vi "Update Value.vi"(6 "Time":dbl, 8 "error in (no error)":errorcluster, 11 "BooleanIndicator in":refnum<class "BooleanIndicator.lvclass">) -> (0 "error out":errorcluster, 1 "Update":bool, 2 "Value":variant, 3 "BooleanIndicator out":refnum<class "BooleanIndicator.lvclass">)   [LabVIEW 2020, in "VolatusGUIElements.lvlib" / "BooleanIndicator.lvclass"]
uses:
  BooleanIndicator.lvclass
  BooleanIndicator.lvclass/BooleanIndicator.ctl
  lv-vecto/Vecto/Channel DBL/Channel DBL.lvclass/Channel DBL.ctl
  lv-vecto/Vecto/Group DBL/Value by Index.vi
  lv-vecto/Vecto/Channel DBL/Channel DBL.lvclass
  lv-vecto/Vecto/Vecto.lvlib
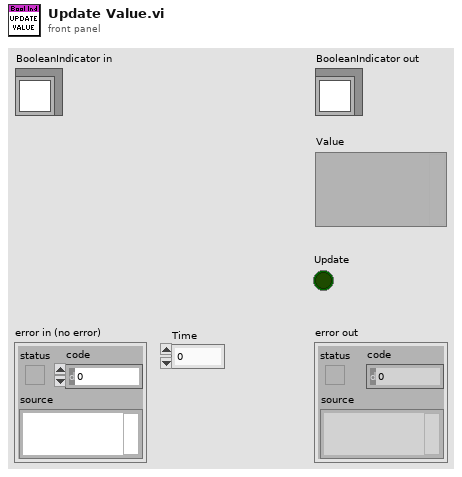
[diagram p1: front panel]
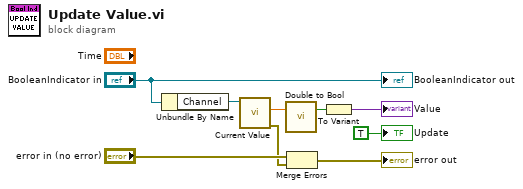
[diagram p0: block diagram]
diagram:
  n1 = Unbundle By Name("BooleanIndicator in") -> ("Channel"=w8:refnum<class "Channel DBL.lvclass">)
  n2 = call "Current Value.vi"("Channel in"=w8) -> ("error out"=w1:errorcluster, "Scaled"=w7:dbl)  [unwired: 6 in, 3 out]
  n3 = call "Double to Bool.vi"("Double"=w7) -> ("Bool"=w5:bool)  [unwired: 2 in]
  n4 = Merge Errors("error in (no error)", w1) -> (→"error out":errorcluster)
  n5 = To Variant(anything=w5) -> (Variant=→"Value":variant)
  "BooleanIndicator out" <- "BooleanIndicator in"
  "Update" <- TRUE ("Update")
